vi "2D binning speed test.vi"() -> ()   [LabVIEW 2018]
uses:
  SubVi's/Controls/CTL_2D_bins_parameters.ctl
  SubVi's/Calc and data manipulation/GET_2D_Data_Binning_(additional_data).vi
  <vilib>/ptbypt/NI_PtbyPt.lvlib
  <vilib>/Analysis/NI_AALBase.lvlib
  Tracker.lvlib
panel:
  out "ms per hour":dbl
  in  "Multiplier":dbl=25.0 format="%#_13g"
  out "X Histogram Graph":T1(graph)
  out "XY binned data":dbl[][](array[numeric])
  in  "SD Y":dbl=1.0 format="%#_13g"
  in  "SD X":dbl=1.0 format="%#_13g"
  in  "N points":i32=360000
  in  "Bins parameters":T2={"Xmax"=110.0, "Xmin"=-110.0, "Ymax"=110.0, "Ymin"=-110.0, "# bins per axis"=11}
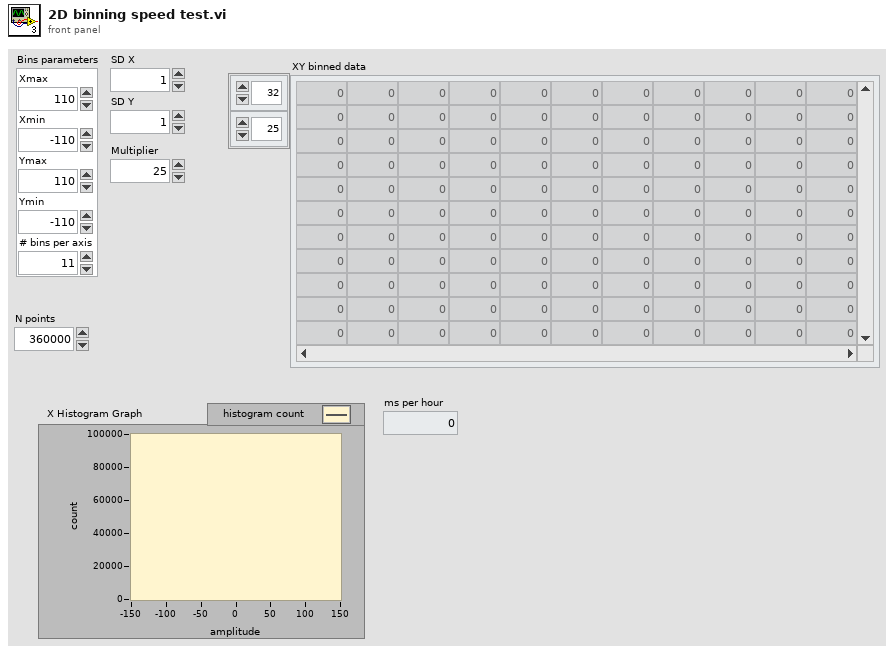
[diagram p1: front panel]
types:
  T1 = cluster{"X Values":dbl[], "Histogram: h(x)":i32[]}
  T2 = typedef "Tracker.lvlib/CTL_2D_bins_parameters.ctl" = cluster{"Xmax":dbl, "Xmin":dbl, "Ymax":dbl, "Ymin":dbl, "# bins per axis":i32}
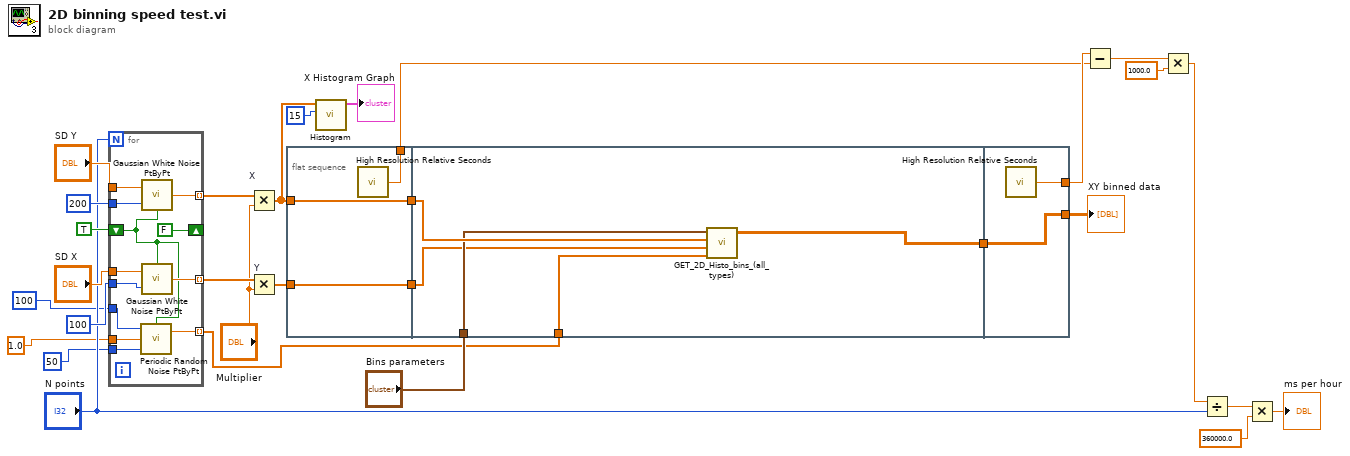
[diagram p0: block diagram]
diagram:
  n1 = for {
    N: "N points" -> [_]
    tunnel: 100 ("seed") -> [w42]
    tunnel: "SD X" -> [w41]
    shift-right: [FALSE] -> _
    shift-left: TRUE -> [w32]
    tunnel: [w39] -> w25 mode=indexing
    tunnel: 200 ("seed") -> [w38]
    tunnel: "SD Y" -> [w37]
    tunnel: [w36] -> w23 mode=indexing
    tunnel: 50 ("seed") -> [w35]
    tunnel: 1.0 ("spectral amplitude") -> [w34]
    tunnel: [w33] -> w1 mode=indexing
    tunnel: 100 ("sample length") -> [w31]
    n2 = call <vilib>:"Periodic Random Noise PtByPt.vi"("initialize"=w32, "seed"=w35, "spectral amplitude"=w34, "sample length"=w31) -> ("periodic random noise"=w33:dbl)  [unwired: 1 out]
    n3 = call <vilib>:"Gaussian White Noise PtByPt.vi"("initialize"=w32, "seed"=w38, "standard deviation"=w37) -> ("Gaussian white noise"=w36:dbl)
    n4 = call <vilib>:"Gaussian White Noise PtByPt.vi"("initialize"=w32, "seed"=w42, "standard deviation"=w41) -> ("Gaussian white noise"=w39:dbl)
  }
  n5 = Multiply "X"(x=w23, y="Multiplier") -> (x*y=w21:dbl[])
  n6 = Multiply "Y"(x=w25, y="Multiplier") -> (x*y=w20:dbl[])
  n7 = flat-sequence {
    tunnel: w20 -> [w44]
    tunnel: w21 -> [w45]
    tunnel: [w45] -> w18
    tunnel: [w44] -> w17
    tunnel: [w43] -> w15
    tunnel: w18 -> [w50]
    tunnel: w17 -> [w48]
    tunnel: "Bins parameters" -> [w49]
    tunnel: [w47] -> w5
    tunnel: w1 -> [w46]
    tunnel: [w52] -> w16
    tunnel: [w51] -> w6
    tunnel: w5 -> [w51]
    frame #0 {
      n8 = call <vilib>:"High Resolution Relative Seconds.vi"() -> ("relative seconds"=w43:dbl)
    }
    frame #1 {
      n9 = call-poly "GET_2D_Histo_bins_(all_types).vi"("Additional data"=w46, "Y"=w48, "X"=w50, "Bins parameters"=w49) -> ("Binned array"=w47:dbl[][])  [unwired: 2 in]
    }
    frame #2 {
      n10 = call <vilib>:"High Resolution Relative Seconds.vi"() -> ("relative seconds"=w52:dbl)
    }
  }
  n11 = call <vilib>:"Histogram.vi"("intervals"=15, "X"=w21) -> ("Histogram Graph"=→"X Histogram Graph":T1)  [unwired: 6 in, 3 out]
  n12 = Subtract(x=w16, y=w15) -> (x-y=w14:dbl)
  n13 = Multiply(x=w14, y=1000.0) -> (x*y=w12:dbl)
  n14 = Divide(x=w12, y="N points") -> (x/y=w10:dbl)
  n15 = Multiply(x=w10, y=360000.0) -> (x*y=→"ms per hour":dbl)
  "XY binned data" <- w6
